vi "Rotational Addition.vi"(0 "Motor 1 in":dbl, 5 "Motor 2 in":dbl, 7 "Motor 3 in":dbl, 9 "Motor 4 in":dbl, 11 "error in":errorcluster, 12 "Rot spd multiplier":dbl=1.0) -> (4 "Motor 1 out":dbl, 6 "Motor 2 out":dbl, 8 "Motor 3 out":dbl, 10 "Motor 4 out":dbl, 15 "error out":errorcluster)   [LabVIEW 2017]
panel:
  # "VI Description: Adds a rotational component to the motors given a speed multiplier"
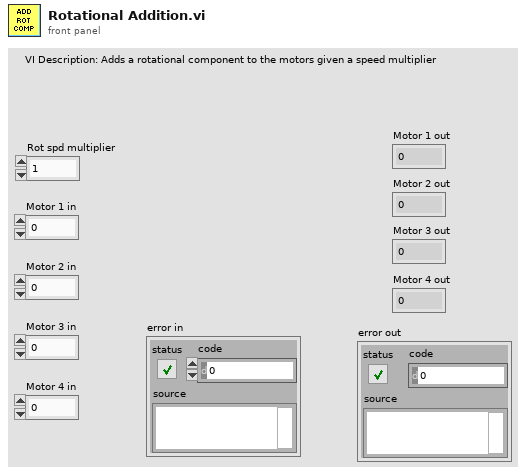
[diagram p1: front panel]
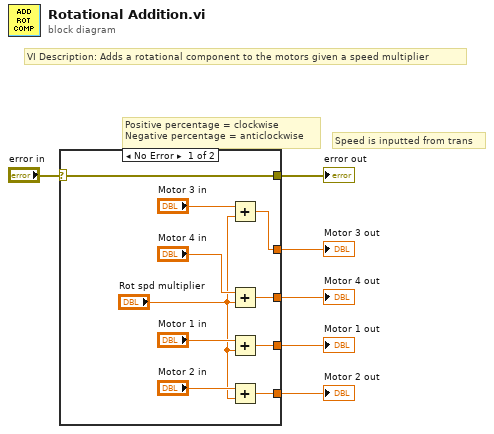
[diagram p0: block diagram]
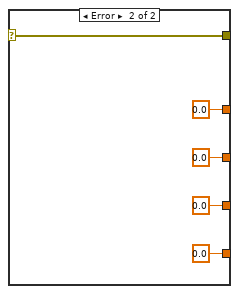
[diagram p2: hidden frame]
diagram:
  # "VI Description: Adds a rotational component to the motors given a speed multiplier"
  # "Positive percentage = clockwise\nNegative percentage = anticlockwise"
  # "Speed is inputted from trans"
  n1 = case shown="No Error" "error in" {
    selector: "error in" -> [w12 w21]
    tunnel: [w12 w21] -> w5
    tunnel: [w10 0.0] -> w4
    tunnel: [w9 0.0] -> w3
    tunnel: [w8 0.0] -> w2
    tunnel: [w7 0.0] -> w1
    frame No Error {
      n2 = Add(x="Motor 3 in", y="Rot spd multiplier") -> (x+y=w9:dbl)
      n3 = Add(x="Motor 4 in", y="Rot spd multiplier") -> (x+y=w8:dbl)
      n4 = Add(x="Motor 1 in", y="Rot spd multiplier") -> (x+y=w7:dbl)
      n5 = Add(x="Motor 2 in", y="Rot spd multiplier") -> (x+y=w10:dbl)
    }
    frame Error {
    }
  }
  "error out" <- w5
  "Motor 2 out" <- w4
  "Motor 3 out" <- w3
  "Motor 4 out" <- w2
  "Motor 1 out" <- w1
